vi "Clear Low Soil Moisture Alarm V.vi"(8 "error in (no error)":errorcluster, 11 "sensorNumber":i32) -> (0 "error out":errorcluster, 3 "function return":i16)   [LabVIEW 2009, in "VantagePro.lvlib"]
doc: "DllAccess short int _stdcall ClearLowSoilMoistureAlarm_V ( int sensorNumber );"
uses:
  VantagePro.lvlib
  <userlib>/VantagePro/VantagePro.dll
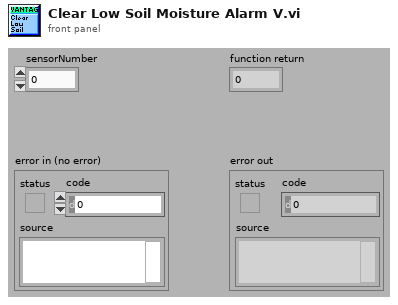
[diagram p1: front panel]
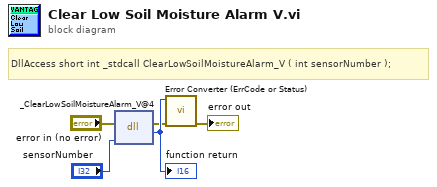
[diagram p0: block diagram]
diagram:
  # "DllAccess short int _stdcall ClearLowSoilMoistureAlarm_V ( int sensorNumber );"
  n1 = dll-call lib="C:/Program Files/National Instruments/LabVIEW 2010/user.lib/VantagePro/VantagePro.*" fn="_ClearLowSoilMoistureAlarm_V@4"(error in="error in (no error)", "sensorNumber"="sensorNumber") -> (error out=w2:errorcluster, w5:i16)  [unwired: 3 in, 1 out]
  "function return" <- w5
  n2 = call "Error Converter (ErrCode or Status).vi"("error in (no error)"=w2, "error code"=w5) -> ("error out"=→"error out":errorcluster)  [unwired: 9 in]
